vi "Empty Key value dialogue.vi"(6 "Type":T1, 7 "Key":string, 9 "Which file or folder?":T2=enum."Calibration Files", 11 "Key's value in":string) -> (1 "Cancel":bool, 3 "Key's value out":string)   [LabVIEW 2013]
uses:
  Typedefs/Which path.ctl
  Typedefs/File or Folder path or name.ctl
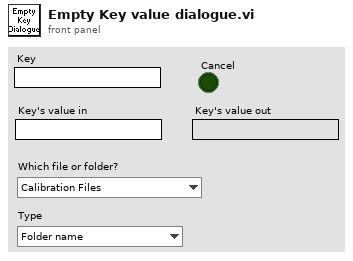
[diagram p1: front panel]
types:
  T1 = typedef "File or Folder path or name.ctl" = enum16{"Folder name", "Folder path", "File name", "File path & name"}
  T2 = typedef "Which path.ctl" = enum16{"Configuration Files", "Calibration Files", "Images", "Setup.ini", "Loaded User profile.ini", "User's-Previous session.ini", "New user profile.ini", "Selected User profile.ini", "User profiles folder", "Power meter scaling.txt", "FOV Cal.ini"}
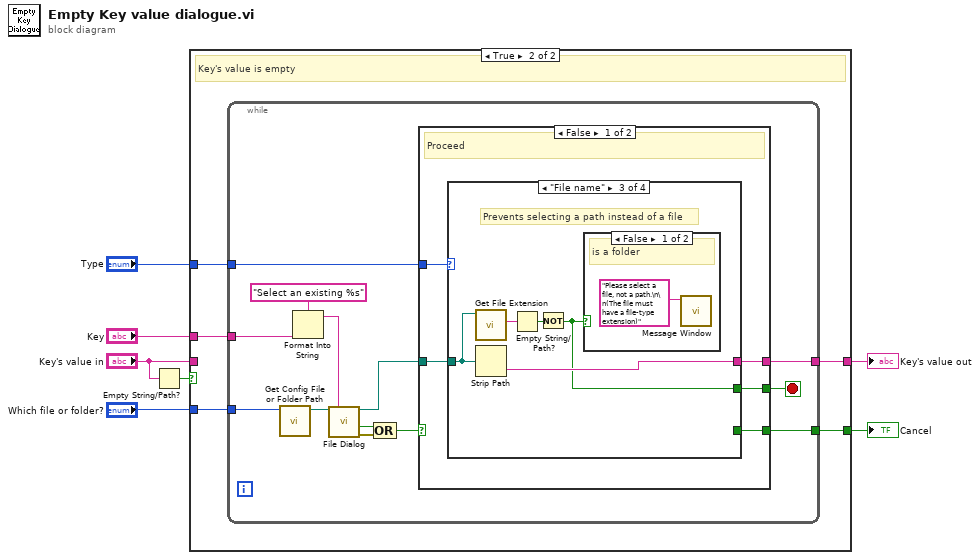
[diagram p0: block diagram]
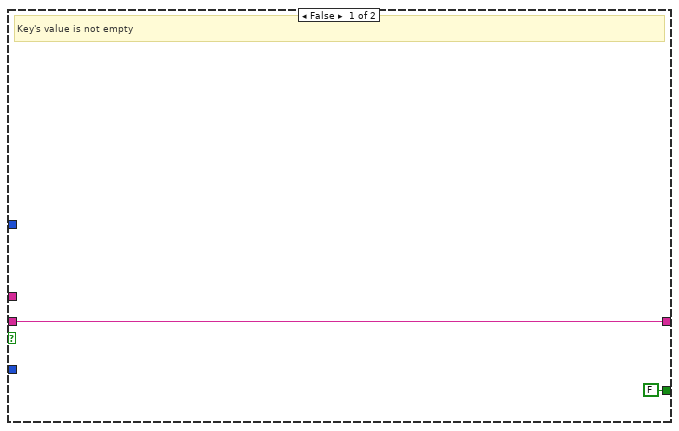
[diagram p2: hidden frame]
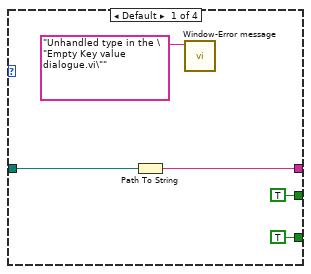
[diagram p3: hidden frame]
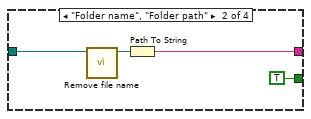
[diagram p4: hidden frame]
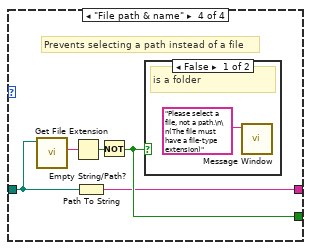
[diagram p6: hidden frame]
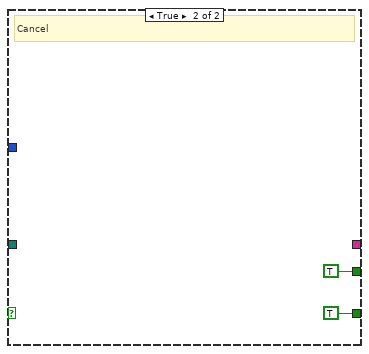
[diagram p8: hidden frame]
diagram:
  n1 = Empty String/Path?(string/path="Key's value in") -> (empty?=w6:bool)
  n2 = case shown="True" w6 {
    tunnel: [w9 w10] -> w7
    tunnel: "Key's value in" -> [w9 _]
    tunnel: "Which file or folder?" -> [_ w14]
    tunnel: "Key" -> [_ w12]
    tunnel: [FALSE w13] -> w2
    tunnel: "Type" -> [_ w11]
    frame False {
      # "Key's value is not empty"
    }
    frame True {
      # "Key's value is empty"
      n3 = while {
        tunnel: w14 -> [w27]
        tunnel: [w15] -> w13
        tunnel: w12 -> [w22]
        tunnel: w11 -> [w20]
        tunnel: [w18] -> w10
        stop <- w17 stop-if-true
        n4 = call "Get Config File or Folder Path.vi"("Which file or folder?"=w27) -> ("File Path"=w26:path)  [unwired: 8 in, 2 out]
        n5 = Format Into String(format string="Select an existing %s" ("prompt"), w22) -> (resulting string=w21:string)  [unwired: 2 in, 1 out]
        n6 = call "File Dialog"("start path"=w26, "prompt"=w21) -> ("selected path"=w19:path, "cancelled"=w24:bool, "error out"=w25:errorcluster)  [unwired: 10 in, 1 out]
        n7 = Compound Arithmetic op=OR(w24, w25) -> (w16:bool)
        n8 = case shown="False" w16 {
          tunnel: w20 -> [w32 _]
          tunnel: w19 -> [w31 _]
          tunnel: [w30 _] -> w18
          tunnel: [w29 TRUE] -> w17
          tunnel: [w28 TRUE] -> w15
          frame False {
            # "Proceed"
            n9 = case shown="\"File name\"" w32 {
              tunnel: w31 -> [w37 w41 w44 w49]
              tunnel: [w36 w39 w43 w48] -> w30
              tunnel: [TRUE TRUE w42 w50] -> w29
              tunnel: [TRUE _ _ _] -> w28
              frame Default {
                n10 = Path To String(path=w37) -> (string=w36:string)
                n11 = call "Window-Error message.vi"("Message"="Unhandled type in the \"Empty Key value dialogue.vi\"") -> ()  [unwired: 10 in, 1 out]
              }
              frame "Folder name", "Folder path" {
                n12 = call "Remove file name.vi"("Input path"=w41) -> ("Path with file name removed"=w40:path)  [unwired: 10 in]
                n13 = Path To String(path=w40) -> (string=w39:string)
              }
              frame "File name" {
                # "Prevents selecting a path instead of a file"
                n14 = call <vilib>:"Get File Extension.vi"("file"=w44) -> ("lowercase file extension"=w46:string)  [unwired: 7 in, 3 out]
                n15 = Strip Path(path=w44) -> (name=w43:string)  [unwired: 1 out]
                n16 = Empty String/Path?(string/path=w46) -> (empty?=w45:bool)
                n17 = Not(x=w45) -> (.not. x?=w42:bool)
                n18 = case shown="False" w42 {
                  frame False {
                    # "is a folder"
                    n19 = call "Message Window.vi"("Message string"="Please select a file, not a path.\n\n(The file must have a file-type extension)") -> ()  [unwired: 10 in, 1 out]
                  }
                  frame True {
                    # "is a file"
                  }
                }
              }
              frame "File path & name" {
                # "Prevents selecting a path instead of a file"
                n20 = call <vilib>:"Get File Extension.vi"("file"=w49) -> ("lowercase file extension"=w52:string)  [unwired: 7 in, 3 out]
                n21 = Empty String/Path?(string/path=w52) -> (empty?=w51:bool)
                n22 = Path To String(path=w49) -> (string=w48:string)
                n23 = Not(x=w51) -> (.not. x?=w50:bool)
                n24 = case shown="False" w50 {
                  frame False {
                    # "is a folder"
                    n25 = call "Message Window.vi"("Message string"="Please select a file, not a path.\n\n(The file must have a file-type extension)") -> ()  [unwired: 10 in, 1 out]
                  }
                  frame True {
                    # "is a file"
                  }
                }
              }
            }
          }
          frame True {
            # "Cancel"
          }
        }
      }
    }
  }
  "Key's value out" <- w7
  "Cancel" <- w2
